vi "Backup LabVIEW.ini File.vi"(8 "error in (no error)":errorcluster) -> (0 "error out":errorcluster, 3 "new path":path)   [LabVIEW 2017]
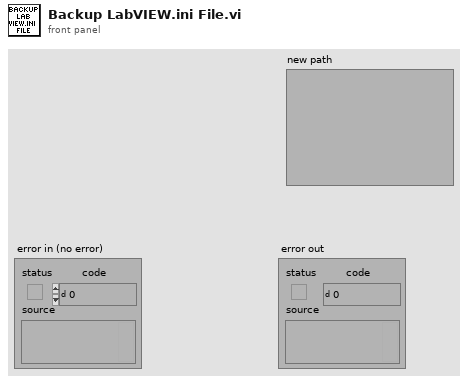
[diagram p1: front panel]
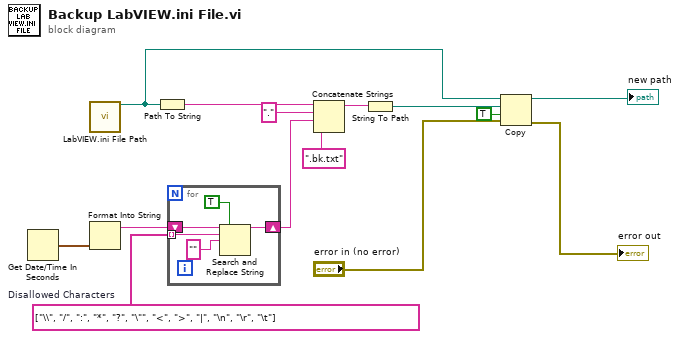
[diagram p0: block diagram]
diagram:
  w4 = string[] ["\\", "/", ":", "*", "?", "\"", "<", ">", "|", "\n", "\r", "\t"]  # Disallowed Characters
  n1 = Get Date/Time In Seconds() -> (seconds since 1Jan1904=w6:timestamp)
  n2 = call "LabVIEW.ini File Path.vi"() -> ("appended path"=w11:path)  [unwired: 19 in]
  n3 = Format Into String(w6) -> (resulting string=w3:string)  [unwired: 3 in, 1 out]
  n4 = Path To String(path=w11) -> (string=w14:string)
  n5 = for {
    tunnel: w4 -> [w17] mode=indexing
    shift-right: [w15] -> w2
    shift-left: w3 -> [w18]
    n6 = Search and Replace String(replace all?=TRUE ("replace all? (F)"), input string=w18, search string=w17, replace string="" ("replace string (\"\")")) -> (result string=w15:string)  [unwired: 4 in, 3 out]
  }
  n7 = Concatenate Strings(w14, "." ("string"), w2, ".bk.txt" ("string")) -> (w12:string)
  n8 = String To Path(string=w12) -> (path=w10:path)
  n9 = Copy(8:"error in (no error)", 9:TRUE ("overwrite (F)"), 10:w10, 11:w11) -> (0:→"error out":errorcluster, 3:→"new path":path)  [unwired: 1 in, 1 out]
